vi "AO Channel.vi"(8 "error in (no error)":errorcluster, 11 "Node Ptr":T1 format="%.0x") -> (0 "error out":errorcluster)   [LabVIEW 2023, in "Waveform Analog Output System Explorer.lvlib"]
uses:
  Waveform Analog Output System Explorer.lvlib
  <vilib>/NI VeriStand/Custom Device API/Custom Device Item Ref.ctl
  Shared/Constants.vi
  <vilib>/NI VeriStand/Custom Device API/Get Item Property (Variant).vi
  <vilib>/NI VeriStand/Custom Device API/Custom Device API.lvlib
  Shared/Waveform Analog Output Shared.lvlib
panel:
  out "DAQ Physical Channel":string
  in  "Header":cluster{"Section Name":string}={"Section Name"="Analog Output Channel"}
  in  "Description":string
  in  "Name":string
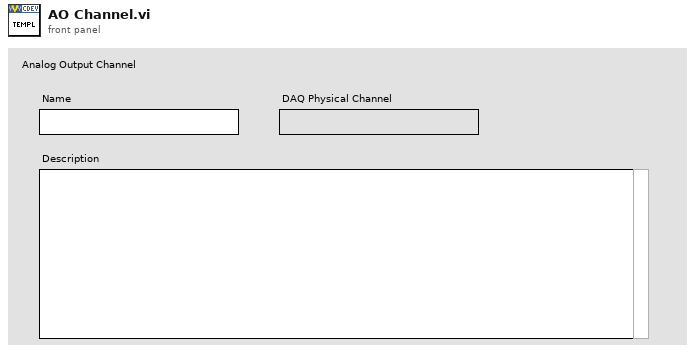
[diagram p1: front panel]
types:
  T1 = typedef "Custom Device API.lvlib/Custom Device Item Ref.ctl" = u64
  T2 = typedef "Custom Device API.lvlib/Custom Device Item Info.ctl" = cluster{"Name":string, "Is Channel":bool, "GUID":string, "Is Waveform":bool}
  T3 = typedef "Custom Device API.lvlib/Custom Device Commands.ctl" = enum16{"Default", "Item renamed", "Shutdown", "Dynamic button pressed"}
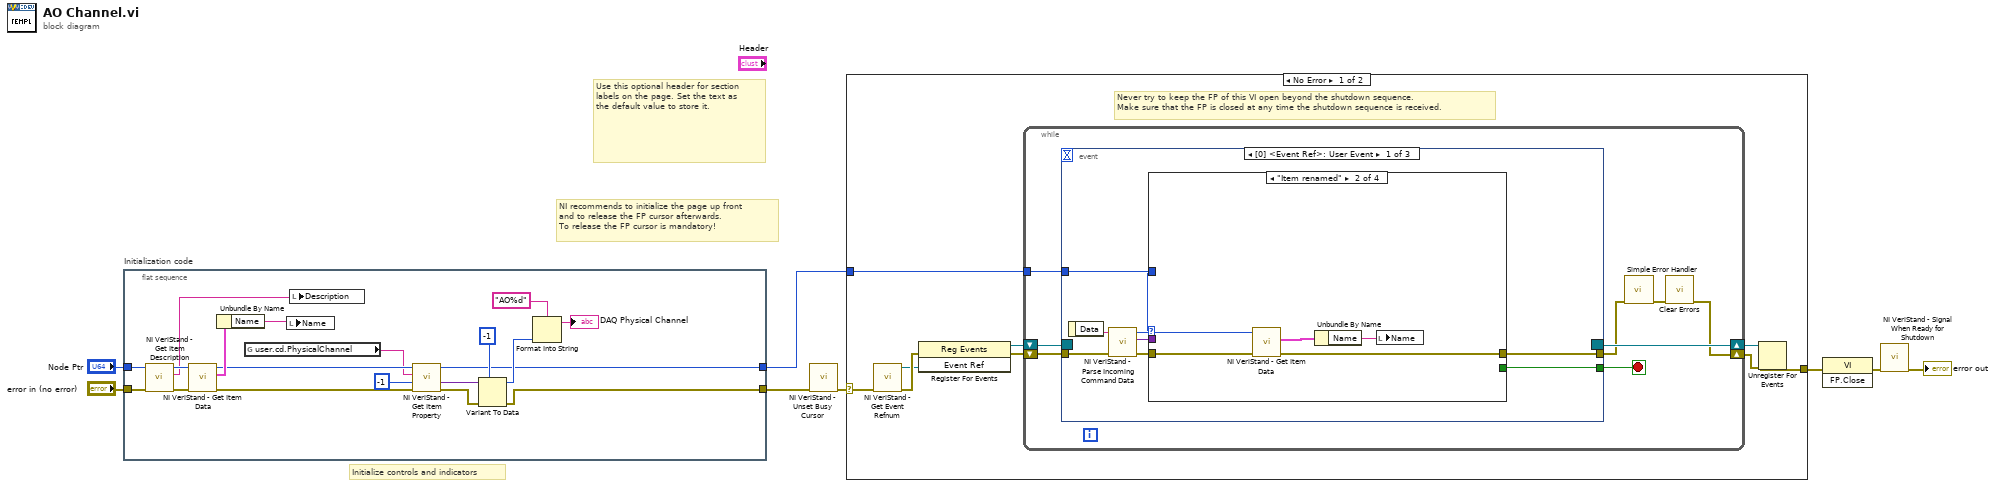
[diagram p0: block diagram]
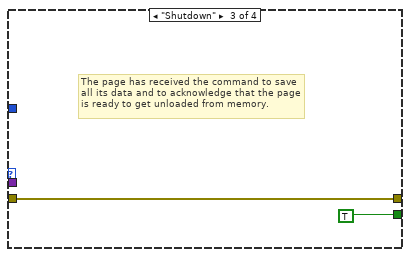
[diagram p3: hidden frame]
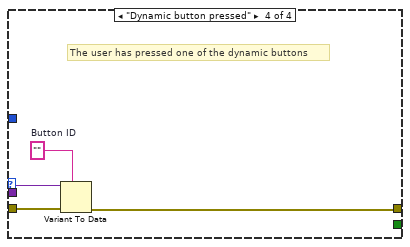
[diagram p4: hidden frame]
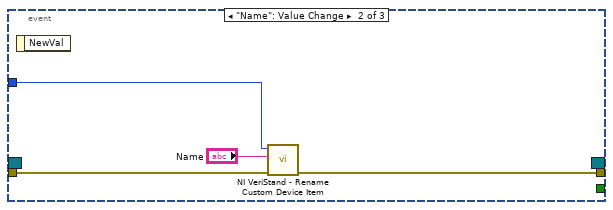
[diagram p5: hidden frame]
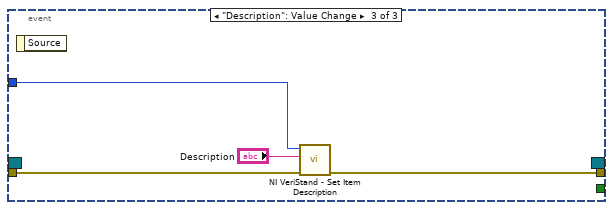
[diagram p6: hidden frame]
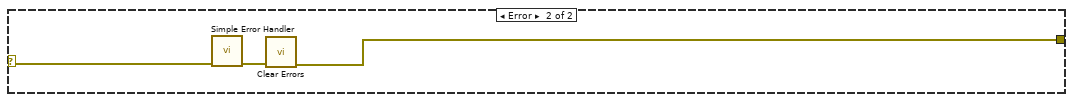
[diagram p7: hidden frame]
diagram:
  # "Initialize controls and indicators"
  # "Use this optional header for section labels on the page. Set the text as the default value to store it."
  # "NI recommends to initialize the page up front\nand to release the FP cursor afterwards.\nTo release the FP cursor is mandatory!"
  n1 = flat-sequence "Initialization code" {
    tunnel: "error in (no error)" -> [w26]
    tunnel: "Node Ptr" -> [w25]
    tunnel: [w12] -> w4
    tunnel: [w11] -> w1
    frame #0 {
      n2 = call <vilib>:"NI VeriStand - Get Item Description.vi"("error in (no error)"=w26, "Item Ref in"=w25) -> ("error out"=w24:errorcluster, "Description"=w9:string, "Item Ref out"=w27:T1)  [unwired: 7 out]
      n3 = call <vilib>:"NI VeriStand - Get Item Data.vi"("error in (no error)"=w24, "Item Ref in"=w27) -> ("error out"=w21:errorcluster, "Item Info"=w23:T2, "Item Ref out"=w22:T1)  [unwired: 7 out]
      n4 = Unbundle By Name(w23) -> ("Name"=w10:string)
      n5 = global read "Constants.vi" "user.cd.PhysicalChannel"() -> (w20:string)
      n6 = local write "Name"(w10) -> ()
      n7 = local write "Description"(w9) -> ()
      n8 = call-poly <vilib>:"NI VeriStand - Get Item Property.vi"("error in (no error)"=w21, "Default Value"=-1, "Property Name"=w20, "Item Ref in"=w22) -> ("error out"=w17:errorcluster, "Value"=w18:variant, "Item Ref out"=w11:T1)  [unwired: 4 in, 1 out]
      n9 = Variant To Data(error in=w17, type=-1, Variant=w18) -> (data=w15:i32, error out=w12:errorcluster)
      n10 = Format Into String(format string="AO%d", w15) -> (resulting string=→"DAQ Physical Channel":string)  [unwired: 2 in, 1 out]
    }
  }
  n11 = call <vilib>:"NI VeriStand - Unset Busy Cursor.vi"("error in (no error)"=w4) -> ("error out"=w3:errorcluster)  [unwired: 10 out]
  n12 = case shown="No Error" w3 {
    selector: w3 -> [w28 w75]
    tunnel: [w33 w73] -> w8
    tunnel: w1 -> [w29 _]
    frame No Error {
      # "Never try to keep the FP of this VI open beyond the shutdown sequence.\nMake sure that the FP is closed at any time the shutdown sequence is received."
      n13 = call <vilib>:"NI VeriStand - Get Event Refnum.vi"("error in (no error)"=w28) -> ("error out"=w36:errorcluster, "Event Ref"=w32:refnum<user-event>)  [unwired: 9 out]
      n14 = register-events(error in=w36, w32) -> (reference out=w30:refnum<event-registration>, error out=w31:errorcluster)  [unwired: 1 in]
      n15 = while {
        tunnel: w29 -> [w40]
        shift-right: [w37] -> w34
        shift-left: w31 -> [w43]
        shift-right: [w44] -> w35
        shift-left: w30 -> [w42]
        stop <- w41 stop-if-true
        n16 = event shown="[0] <Event Ref>: User Event" {
          selector: w42 -> [_ _ _]
          dyn-events: [_ _ _] -> w44
          timeout: _ -> [_ _ _]
          tunnel: w43 -> [w52 w68 w71]
          tunnel: [w48 _ _] -> w41
          tunnel: [w47 w67 w70] -> w39
          tunnel: w40 -> [w46 w66 w72]
          event User Event {
            n17 = event-data() -> ("Data"=w51:string)  [unwired: 1 out]
            n18 = call <vilib>:"NI VeriStand - Parse Incoming Command Data.vi"("error in (no error)"=w52, "Incoming data"=w51) -> ("error out"=w50:errorcluster, "Outgoing data"=w45:variant, "Action"=w49:T3)  [unwired: 7 out]
            n19 = case shown="\"Item renamed\"" w49 {
              tunnel: w50 -> [w53 w58 w59 w64]
              tunnel: [_ _ TRUE _] -> w48
              tunnel: [w53 w55 w59 w61] -> w47
              tunnel: w46 -> [_ w57 _ _]
              tunnel: w45 -> [_ _ _ w63]
              frame "Default", Default {
              }
              frame "Item renamed" {
                n20 = call <vilib>:"NI VeriStand - Get Item Data.vi"("error in (no error)"=w58, "Item Ref in"=w57) -> ("error out"=w55:errorcluster, "Item Info"=w56:T2)  [unwired: 8 out]
                n21 = Unbundle By Name(w56) -> ("Name"=w54:string)
                n22 = local write "Name"(w54) -> ()
              }
              frame "Shutdown" {
                # "The page has received the command to save all its data and to acknowledge that the page is ready to get unloaded from memory."
              }
              frame "Dynamic button pressed" {
                w62 = ""  # Button ID
                # "The user has pressed one of the dynamic buttons"
                n23 = Variant To Data(error in=w64, type=w62, Variant=w63) -> (error out=w61:errorcluster)  [unwired: 1 out]
              }
            }
          }
          event "Name": Value Change {
            n24 = event-data() -> ()  [unwired: 2 out]
            n25 = call <vilib>:"NI VeriStand - Rename Custom Device Item.vi"("error in (no error)"=w68, "New Name"="Name", "Item Ref in"=w66) -> ("error out"=w67:errorcluster)  [unwired: 1 in, 7 out]
          }
          event "Description": Value Change {
            n26 = event-data() -> ()  [unwired: 2 out]
            n27 = call <vilib>:"NI VeriStand - Set Item Description.vi"("error in (no error)"=w71, "Description"="Description", "Item Ref in"=w72) -> ("error out"=w70:errorcluster)  [unwired: 8 out]
          }
        }
        n28 = call <vilib>:"Simple Error Handler.vi"("error in (no error)"=w39) -> ("error out"=w38:errorcluster)  [unwired: 1 in, 7 out]
        n29 = call <vilib>:"Clear Errors.vi"("error in (no error)"=w38) -> ("error out"=w37:errorcluster)  [unwired: 1 in, 5 out]
      }
      n30 = Unregister For Events(event registration refnum=w35, error in=w34) -> (error out=w33:errorcluster)
    }
    frame Error {
      n31 = call <vilib>:"Simple Error Handler.vi"("error in (no error)"=w75) -> ("error out"=w74:errorcluster)  [unwired: 1 in, 7 out]
      n32 = call <vilib>:"Clear Errors.vi"("error in (no error)"=w74) -> ("error out"=w73:errorcluster)  [unwired: 1 in, 5 out]
    }
  }
  n33 = invoke class="VI" method="FP.Close"(error in=w8) -> (error out=w7:errorcluster)  [unwired: 2 in, 2 out]
  n34 = call <vilib>:"NI VeriStand - Signal When Ready for Shutdown.vi"("error in (no error)"=w7) -> ("error out"=→"error out":errorcluster)  [unwired: 10 out]
